vi "X10468 SLM Load Flat File.vi"(7 "Flat File Path":path, 11 "Error In":errorcluster) -> (4 "Selected File":path, 8 "SLM Flat Map":dbl[][](array[numeric]), 15 "Error Out":errorcluster)   [LabVIEW 2018]
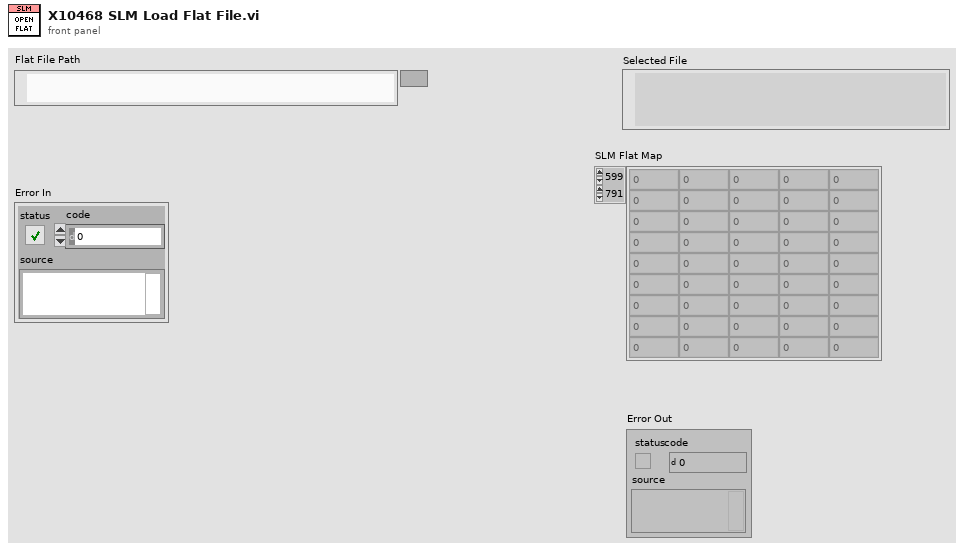
[diagram p1: front panel]
types:
  T1 = typedef "IMAQ Image.ctl" = refnum<image>
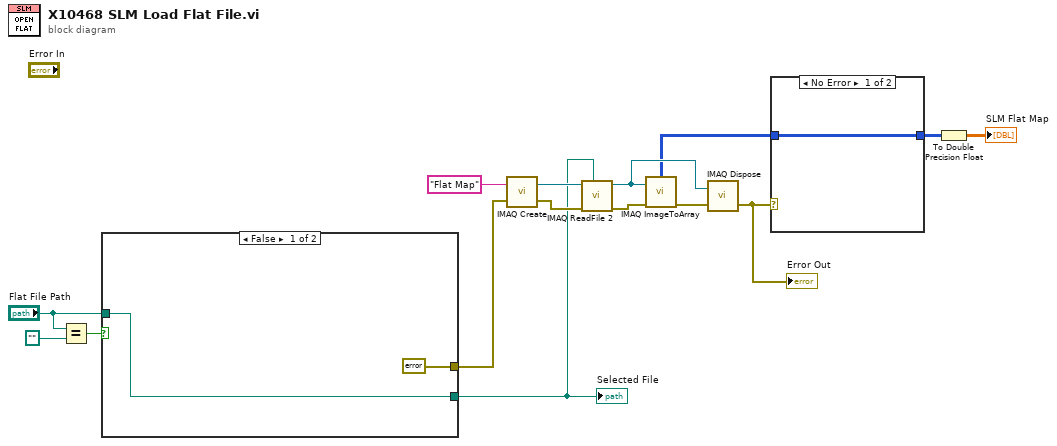
[diagram p0: block diagram]
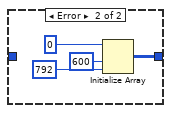
[diagram p2: hidden frame]
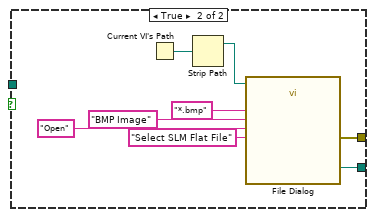
[diagram p3: hidden frame]
diagram:
  n1 = Equal?(x="Flat File Path", y=path "") -> (x = y?=w8:bool)
  n2 = case shown="False" w8 {
    tunnel: [w16 w19] -> w6
    tunnel: [errorcluster {"status"=FALSE, "code"=0, "source"=""} ("error out") w18] -> w7
    tunnel: "Flat File Path" -> [w16 _]
    frame False {
    }
    frame True {
      n3 = Current VI's Path() -> (path=w25:path)
      n4 = Strip Path(path=w25) -> (stripped path=w24:path)  [unwired: 1 out]
      n5 = call "File Dialog"("start path"=w24, "prompt"="Select SLM Flat File", "button label"="Open", "pattern (all files)"="*.bmp", "pattern label"="BMP Image") -> ("selected path"=w19:path, "error out"=w18:errorcluster)  [unwired: 7 in, 2 out]
    }
  }
  "Selected File" <- w6
  n6 = call "IMAQ Create"("Image Name"="Flat Map", "error in (no error)"=w7) -> ("New Image"=w14:T1, "error out"=w13:errorcluster)  [unwired: 3 in]
  n7 = call "IMAQ ReadFile 2"("File Path"=w6, "error in (no error)"=w13, "Image"=w14) -> ("error out"=w12:errorcluster, "Image Out"=w10:T1)  [unwired: 4 in, 3 out]
  n8 = call "IMAQ ImageToArray"("error in (no error)"=w12, "Image"=w10) -> ("error out"=w11:errorcluster, "Image Pixels (U8)"=w3:u8[][])  [unwired: 2 in, 3 out]
  n9 = call "IMAQ Dispose"("Image"=w10, "error in (no error)"=w11) -> ("error out"=w4:errorcluster)  [unwired: 4 in]
  "Error Out" <- w4
  n10 = case shown="No Error" w4 {
    tunnel: w3 -> [w26 _]
    tunnel: [w26 w27] -> w2
    frame No Error {
    }
    frame Error {
      n11 = Initialize Array(u8 0 ("element"), 600 ("dimension size"), 792 ("dimension size")) -> (w27:u8[][])
    }
  }
  n12 = To Double Precision Float(number=w2) -> (double precision float=→"SLM Flat Map":dbl[][])
